vi "Obtain Aircraft Queue.vi"(8 "error in (no error)":errorcluster, 11 "Queue Name":string) -> (0 "error out":errorcluster, 3 "queue out":refnum<queue>)   [LabVIEW 2014]
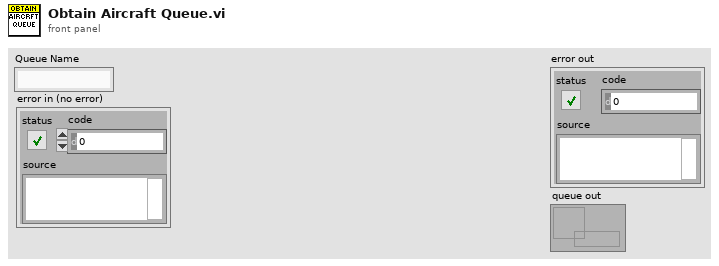
[diagram p1: front panel]
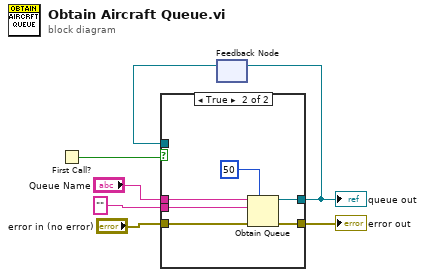
[diagram p0: block diagram]
diagram:
  n1 = First Call?() -> (First Call?: T/F=w3:bool)
  n2 = feedback #1() -> (w1:refnum<queue>)  [unwired: 1 in]
  n3 = case shown="True" w3 {
    tunnel: "Queue Name" -> [_ w15]
    tunnel: "" -> [_ w14]
    tunnel: "error in (no error)" -> [w8 w13]
    tunnel: [w8 w11] -> w4
    tunnel: [w9 w10] -> w2
    tunnel: w1 -> [w9 _]
    frame False {
    }
    frame True {
      n4 = Obtain Queue(max queue size (-1, unlimited)=50, name (unnamed)=w15, element data type=w14, error in (no error)=w13) -> (queue out=w10:refnum<queue>, error out=w11:errorcluster)  [unwired: 1 in, 1 out]
    }
  }
  "error out" <- w4
  "queue out" <- w2
  n5 = feedback-in #1(w2) -> ()
